vi "Get Summary.vi"(10 "Item":string, 11 "Result Model In":refnum<class "Result Model.lvclass">) -> (2 "Summary":string)   [LabVIEW 2020, in "Result Model.lvclass"]
uses:
  Result Model.lvclass
  Result Model.lvclass/Result Model.ctl
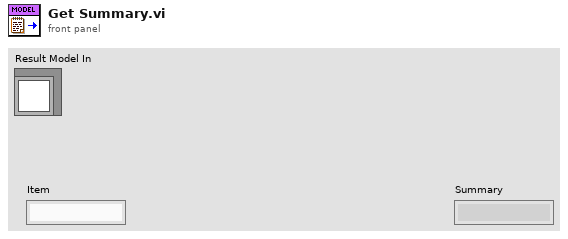
[diagram p1: front panel]
types:
  T1 = typedef "Result Model.lvclass/Model State.ctl" = cluster{"Run Queue":set{string}, "Test Statuses":map{string, T2}, "Execution Time":map{string, dbl}, "Assertions":map{string, cluster{"Result Type":T3, "Status":T2, "Message":string, "Description":string}[]}}
  T2 = typedef "Result.lvlib/Status.ctl" = enum16{"", "Passed", "Failed", "Error", "Skipped", "Setup Error", "Broken", "Teardown Error"}
  T3 = typedef "Result.lvlib/Type.ctl" = enum16{"Method", "Case", "Suite", "Pass", "Fail", "Skip", "Pass if", "Fail if", "Pass if Error", "Fail if Error", "Pass if Equal", "Fail if Equal"}
  T4 = map{string, cluster{"Result Type":T3, "Status":T2, "Message":string, "Description":string}[]}
  T5 = cluster{"Result Type":T3, "Status":T2, "Message":string, "Description":string}[]
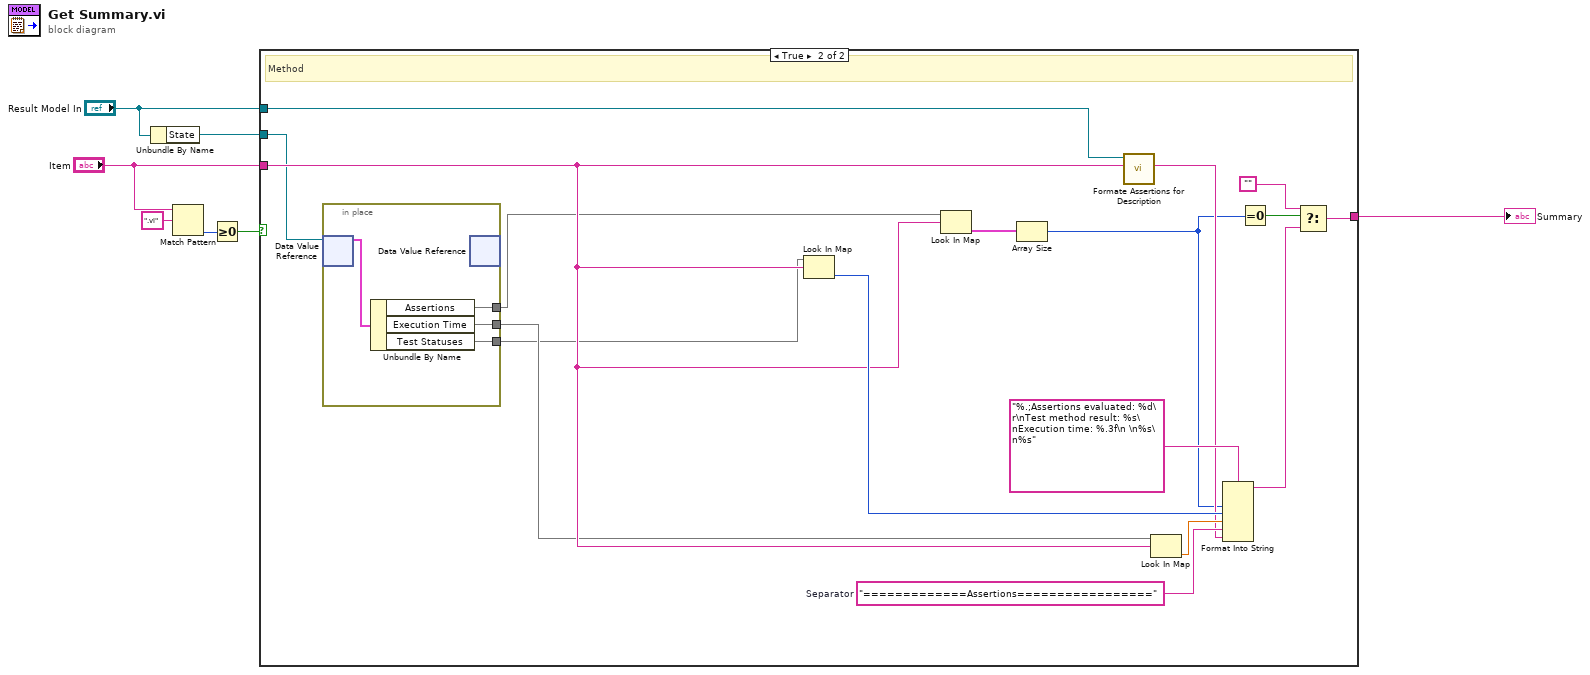
[diagram p0: block diagram]
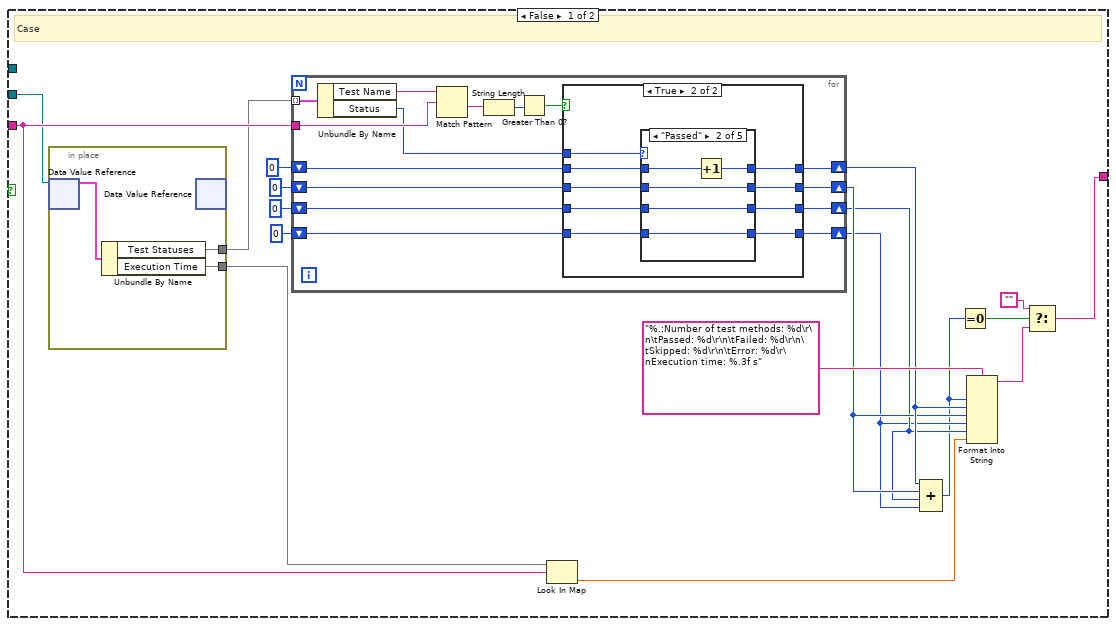
[diagram p2: hidden frame]
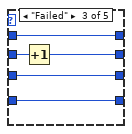
[diagram p5: hidden frame]
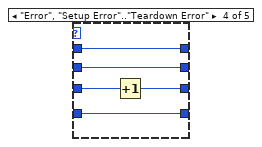
[diagram p6: hidden frame]
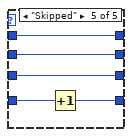
[diagram p7: hidden frame]
diagram:
  n1 = Unbundle By Name("Result Model In") -> ("State"=w1:refnum<data-value>)
  n2 = Match Pattern(string="Item", regular expression=".vi") -> (offset past match=w6:i32)  [unwired: 1 in, 3 out]
  n3 = Greater Or Equal To 0?(x=w6) -> (x >= 0?=w5:bool)
  n4 = case shown="True" w5 {
    tunnel: "Result Model In" -> [_ w94]
    tunnel: "Item" -> [w24 w92]
    tunnel: [w12 w87] -> w3
    tunnel: w1 -> [w10 w85]
    frame False {
      # "Case"
      n5 = in-place {
        in-place-border: [w29] -> w9
        in-place-border: [w28] -> w8
        n6 = in-place-dvr #1(w10) -> (w27:T1)  [unwired: 1 out]
        n7 = Unbundle By Name(w27) -> ("Test Statuses"=w29:map{string, T2}, "Execution Time"=w28:map{string, dbl})
        n8 = in-place-dvr #1() -> ()  [unwired: 1 in, 2 out]
      }
      n9 = for {
        tunnel: w9 -> [w44] mode=indexing
        tunnel: w24 -> [w42]
        shift-right: [w38] -> w22
        shift-left: 0 ("value") -> [w40]
        shift-right: [w36] -> w20
        shift-left: 0 ("value") -> [w37]
        shift-right: [w34] -> w18
        shift-left: 0 ("value") -> [w35]
        shift-right: [w33] -> w16
        shift-left: 0 ("value") -> [w32]
        n10 = Unbundle By Name(w44) -> ("Test Name"=w43:string, "Status"=w41:T2)
        n11 = Match Pattern(string=w43, regular expression=w42) -> (after substring=w31:string)  [unwired: 1 in, 3 out]
        n12 = String Length(string=w31) -> (length=w30:i32)
        n13 = Greater Than 0?(x=w30) -> (x > 0?=w39:bool)
        n14 = case shown="True" w39 {
          tunnel: w41 -> [_ w57]
          tunnel: w40 -> [w48 w56]
          tunnel: [w48 w55] -> w38
          tunnel: w37 -> [w47 w54]
          tunnel: [w47 w53] -> w36
          tunnel: w35 -> [w45 w52]
          tunnel: [w45 w51] -> w34
          tunnel: [w46 w50] -> w33
          tunnel: w32 -> [w46 w49]
          frame False {
          }
          frame True {
            n15 = case shown="\"Passed\"" w57 {
              tunnel: w56 -> [w61 w66 w71 w75 w81]
              tunnel: [w61 w65 w71 w75 w81] -> w55
              tunnel: w54 -> [w60 w64 w70 w76 w80]
              tunnel: [w60 w64 w69 w76 w80] -> w53
              tunnel: w52 -> [w59 w63 w68 w74 w79]
              tunnel: [w59 w63 w68 w73 w79] -> w51
              tunnel: [w58 w62 w67 w72 w77] -> w50
              tunnel: w49 -> [w58 w62 w67 w72 w78]
              frame "" {
              }
              frame "Passed" {
                n16 = Increment(x=w66) -> (x+1=w65:i32)
              }
              frame "Failed" {
                n17 = Increment(x=w70) -> (x+1=w69:i32)
              }
              frame "Error", "Setup Error".."Teardown Error" {
                n18 = Increment(x=w74) -> (x+1=w73:i32)
              }
              frame "Skipped" {
                n19 = Increment(x=w78) -> (x+1=w77:i32)
              }
            }
          }
        }
      }
      n20 = Look In Map(map=w8, key=w24) -> (value=w25:dbl)  [unwired: 1 in, 1 out]
      n21 = Compound Arithmetic op=ADD(w22, w20, w18, w16) -> (w15:i32)
      n22 = Equal To 0?(x=w15) -> (x = 0?=w14:bool)
      n23 = Format Into String(format string="%.;Number of test methods: %d\r\n\tPassed: %d\r\n\tFailed: %d\r\n\tSkipped: %d\r\n\tError: %d\r\nExecution time: %.3f s", w15, w22, w20, w16, w18, w25) -> (resulting string=w13:string)  [unwired: 2 in, 1 out]
      n24 = Select(t="", s=w14, f=w13) -> (s? t:f=w12:string)
    }
    frame True {
      w97 = "=============Assertions================="  # Separator
      # "Method"
      n25 = in-place {
        in-place-border: [w101] -> w84
        in-place-border: [w100] -> w83
        in-place-border: [w99] -> w82
        n26 = in-place-dvr #2(w85) -> (w102:T1)  [unwired: 1 out]
        n27 = Unbundle By Name(w102) -> ("Assertions"=w101:T4, "Execution Time"=w100:map{string, dbl}, "Test Statuses"=w99:map{string, T2})
        n28 = in-place-dvr #2() -> ()  [unwired: 1 in, 2 out]
      }
      n29 = Look In Map(map=w82, key=w92) -> (value=w95:T2)  [unwired: 1 in, 1 out]
      n30 = Look In Map(map=w84, key=w92) -> (value=w91:T5)  [unwired: 1 in, 1 out]
      n31 = Array Size(array=w91) -> (size(s)=w90:i32)
      n32 = call "Formate Assertions for Description.vi"("Item"=w92, "Result Model in"=w94) -> ("Assertions Description"=w93:string)  [unwired: 9 in]
      n33 = Look In Map(map=w83, key=w92) -> (value=w96:dbl)  [unwired: 1 in, 1 out]
      n34 = Format Into String(format string="%.;Assertions evaluated: %d\r\nTest method result: %s\nExecution time: %.3f\n \n%s\n%s", w90, w95, w96, w97, w93) -> (resulting string=w88:string)  [unwired: 2 in, 1 out]
      n35 = Equal To 0?(x=w90) -> (x = 0?=w89:bool)
      n36 = Select(t="", s=w89, f=w88) -> (s? t:f=w87:string)
    }
  }
  "Summary" <- w3
